vi "EncodeMaskedBytes.vi"(8 "error in (no error)":errorcluster, 11 "Raw Data":u8[](array[numeric])) -> (0 "error out":errorcluster, 3 "Masked Data":u8[](array[numeric]))   [LabVIEW 2013, in "WebSockets.lvlib"]
doc: "Unmasks incoming data. Data sent to the client does not need to be masked."
uses:
  WebSockets.lvlib
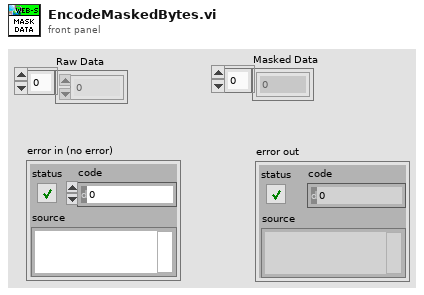
[diagram p1: front panel]
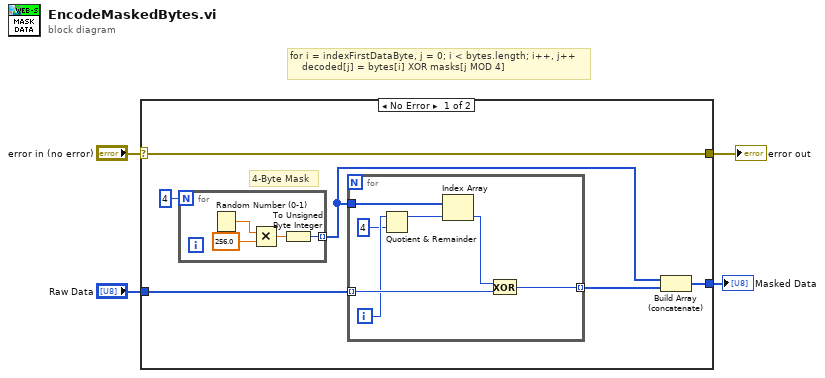
[diagram p0: block diagram]
diagram:
  # "for i = indexFirstDataByte, j = 0; i < bytes.length; i++, j++\n    decoded[j] = bytes[i] XOR masks[j MOD 4]"
  n1 = case shown="No Error" "error in (no error)" {
    selector: "error in (no error)" -> [w10 w22]
    tunnel: [w6 _] -> w2
    tunnel: [w10 w22] -> w3
    tunnel: "Raw Data" -> [w5 _]
    frame No Error {
      # "4-Byte Mask"
      n2 = for {
        N: 4 -> [_]
        tunnel: [w11] -> w8 mode=indexing
        n3 = Random Number (0-1)() -> (number: 0 to 1=w14:dbl)
        n4 = Multiply(x=w14, y=256.0) -> (x*y=w12:dbl)
        n5 = To Unsigned Byte Integer(number=w12) -> (unsigned 8bit integer=w11:u8)
      }
      n6 = for {
        tunnel: w5 -> [w21] mode=indexing
        tunnel: w8 -> [w17]
        tunnel: [w15] -> w7 mode=indexing
        i -> [w20]
        n7 = Quotient & Remainder(x=w20, y=4) -> (x-y*floor(x/y)=w18:i32)  [unwired: 1 out]
        n8 = Index Array(array=w17, index=w18) -> (element=w16:u8)
        n9 = Exclusive Or(1:w21, 2:w16) -> (0:w15:u8)
      }
      n10 = Build Array (concatenate)(w8, w7) -> (w6:u8[])
    }
    frame Error {
    }
  }
  "error out" <- w3
  "Masked Data" <- w2
